vi "Lab Panel V4.86.vi"() -> ()   [LabVIEW 2013] (continued)
        }
        frame #9 {
          # "check network directory valid"
          n212 = while {
            stop <- w260 continue-if-true
            w258 = TRUE
            n213 = local read "Network Directory"() -> (w262:path)
            n214 = property on="Tab Control 2" class="TabCtl (strict)"("Value"=5) -> ()  [unwired: 2 in, 2 out]
            n215 = File/Directory Info(path=w262) -> (error out=w263:errorcluster)  [unwired: 1 in, 6 out]
            n216 = Unbundle(w263) -> ("status"=w260:bool)  [unwired: 2 out]
            n217 = case shown="True" w260 {
              frame False {
                n218 = local write "Message"("") -> ()
              }
              frame True {
                "Message" <- "NETWORK DIRECTORY NOT FOUND!!!!"
              }
            }
            n219 = property on="Message" class="Str"("Text.TextColor"=u32 16711680) -> ()  [unwired: 2 in, 2 out]
            n220 = property on="Network Directory" class="Path"("Blinking"=w258) -> ()  [unwired: 2 in, 2 out]
            n221 = property on="Message" class="Str"("Blinking"=w258) -> ()  [unwired: 2 in, 2 out]
          }
        }
        frame #10 {
          w266 = FALSE
          n222 = property on="Message" class="Str"("Blinking"=w266) -> ()  [unwired: 2 in, 2 out]
          n223 = property on="Network Directory" class="Path"("Blinking"=w266) -> ()  [unwired: 2 in, 2 out]
          n224 = property on="Tab Control 2" class="TabCtl (strict)"("Value"=0) -> ()  [unwired: 2 in, 2 out]
        }
      }
    }
    frame #2 {
      n225 = node-c288("loop  delay(mS)") -> (w270:T15)  [unwired: 3 in]
      n226 = timed-loop {
        timing: w270 -> [_]
        timing-out: [_] -> w269
        i -> [w292]
        stop <- "stop" stop-if-true
        n227 = node-c288() -> ()  [unwired: 1 in, 1 out]
        n228 = global write "Global display 1.vi" "stop disp"("stop") -> ()
        n229 = local read "SELECT LAB05-2"() -> (w272:T3)
        n230 = local read "SELECT LAB05-1"() -> (w273:T3)
        n231 = local read "SELECT LAB04-2"() -> (w274:T3)
        n232 = local read "SELECT LAB03-1"() -> (w277:T3)
        n233 = local read "SELECT LAB02-2"() -> (w278:T3)
        n234 = local read "SELECT LAB01-1"() -> (w281:T3)
        n235 = local read "SELECT LAB03-2"() -> (w276:T3)
        n236 = local read "SELECT LAB01-2"() -> (w280:T3)
        n237 = local read "SELECT LAB04-1"() -> (w275:T3)
        n238 = local read "SELECT LAB02-1"() -> (w279:T3)
        n239 = local read "run lab03-2"() -> (w286:bool)
        n240 = local read "run lab04-1"() -> (w285:bool)
        n241 = local read "run lab05-1"() -> (w283:bool)
        n242 = local read "run lab04-2"() -> (w284:bool)
        n243 = local read "run lab05-2"() -> (w282:bool)
        n244 = local read "run lab03-1"() -> (w287:bool)
        n245 = local read "run lab02-2"() -> (w288:bool)
        n246 = local read "run lab02-1"() -> (w289:bool)
        n247 = local read "run lab01-1"() -> (w291:bool)
        n248 = local read "run lab01-2"() -> (w290:bool)
        n249 = stacked-sequence {
          seq-local: [_ w354 _ _ _ _ _ _ _ _ _ _ _ _ _ _ _ _ _ _ _ _] -> [_ _ _ _ _ w2146 _ _ _ _ _ _ _ _ _ _ _ _ _ _ _ _]
          seq-local: [_ w353 _ _ _ _ _ _ _ _ _ _ _ _ _ _ _ _ _ _ _ _] -> [_ _ _ _ _ w2145 _ _ _ _ _ _ _ _ _ _ _ _ _ _ _ _]
          seq-local: [_ w340 _ _ _ _ _ _ _ _ _ _ _ _ _ _ _ _ _ _ _ _] -> [_ _ _ _ _ w2144 _ _ _ _ _ _ _ _ _ _ _ _ _ _ _ _]
          seq-local: [_ w339 _ _ _ _ _ _ _ _ _ _ _ _ _ _ _ _ _ _ _ _] -> [_ _ _ _ _ w2143 _ _ _ _ _ _ _ _ _ _ _ _ _ _ _ _]
          seq-local: [_ w338 _ _ _ _ _ _ _ _ _ _ _ _ _ _ _ _ _ _ _ _] -> [_ _ _ _ _ w2142 _ _ _ _ _ _ _ _ _ _ _ _ _ _ _ _]
          seq-local: [_ w337 _ _ _ _ _ _ _ _ _ _ _ _ _ _ _ _ _ _ _ _] -> [_ _ _ _ _ w2141 _ _ _ _ _ _ _ _ _ _ _ _ _ _ _ _]
          seq-local: [_ w336 _ _ _ _ _ _ _ _ _ _ _ _ _ _ _ _ _ _ _ _] -> [_ _ _ _ _ w2140 _ _ _ _ _ _ _ _ _ _ _ _ _ _ _ _]
          seq-local: [_ w335 _ _ _ _ _ _ _ _ _ _ _ _ _ _ _ _ _ _ _ _] -> [_ _ _ _ _ w2139 _ _ _ _ _ _ _ _ _ _ _ _ _ _ _ _]
          seq-local: [_ w334 _ _ _ _ _ _ _ _ _ _ _ _ _ _ _ _ _ _ _ _] -> [_ _ _ _ _ w2138 _ _ _ _ _ _ _ _ _ _ _ _ _ _ _ _]
          seq-local: [_ w333 _ _ _ _ _ _ _ _ _ _ _ _ _ _ _ _ _ _ _ _] -> [_ _ _ _ _ w2137 _ _ _ _ _ _ _ _ _ _ _ _ _ _ _ _]
          tunnel: w291 -> [_ _ w370 w612 w1736 w2166 w2481 w2968 _ _ _ _ w3372 _ w4306 _ _ w4591 w4894 w5075 _ _]
          tunnel: w290 -> [_ _ w369 w610 w1735 w2165 w2482 w2967 _ _ _ _ w3371 _ w4304 _ _ w4590 w4893 w5073 _ _]
          tunnel: w289 -> [_ _ w368 w608 w1734 w2164 w2480 w2966 _ _ _ _ w3370 _ w4302 _ _ w4589 w4892 w5072 _ _]
          tunnel: w288 -> [_ _ w367 w606 w1733 w2163 w2479 w2965 _ _ _ _ w3369 _ w4300 _ _ w4588 w4891 w5071 _ _]
          tunnel: w287 -> [_ _ w366 w604 w1732 w2162 w2478 w2964 _ _ _ _ w3368 _ w4298 _ _ w4587 w4890 w5070 _ _]
          tunnel: w286 -> [_ _ w365 w602 w1731 w2161 w2477 w2963 _ _ _ _ w3367 _ w4296 _ _ w4586 w4889 w5069 _ _]
          tunnel: w285 -> [_ _ w364 w600 w1730 w2160 w2476 w2962 _ _ _ _ w3366 _ w4294 _ _ w4585 w4888 w5068 _ _]
          tunnel: w284 -> [_ _ w363 w598 w1729 w2159 w2475 w2961 _ _ _ _ w3365 _ w4292 _ _ w4584 w4887 w5067 _ _]
          tunnel: w283 -> [_ _ w362 w596 w1728 w2158 w2474 w2960 _ _ _ _ w3364 _ w4290 _ _ w4583 w4886 w5066 _ _]
          tunnel: w282 -> [_ _ w361 w594 w1727 w2157 w2473 w2959 _ _ _ _ w3363 _ w4288 _ _ w4582 w4885 w5065 _ _]
          tunnel: w281 -> [_ _ _ w611 w1726 w2156 _ _ _ _ _ _ _ _ w4308 _ _ _ _ _ w5389 _]
          tunnel: w280 -> [_ _ _ w609 w1725 w2155 _ _ _ _ _ _ _ _ w4303 _ _ _ _ _ w5388 _]
          tunnel: w279 -> [_ _ _ w607 w1724 w2154 _ _ _ _ _ _ _ _ w4301 _ _ _ _ _ w5387 _]
          tunnel: w278 -> [_ _ _ w605 w1723 w2153 _ _ _ _ _ _ _ _ w4299 _ _ _ _ _ w5386 _]
          tunnel: w277 -> [_ _ _ w603 w1722 w2152 _ _ _ _ _ _ _ _ w4297 _ _ _ _ _ w5385 _]
          tunnel: w276 -> [_ _ _ w601 w1721 w2151 _ _ _ _ _ _ _ _ w4295 _ _ _ _ _ w5384 _]
          tunnel: w275 -> [_ _ _ w599 w1720 w2150 _ _ _ _ _ _ _ _ w4293 _ _ _ _ _ w5383 _]
          tunnel: w274 -> [_ _ _ w597 w1719 w2149 _ _ _ _ _ _ _ _ w4291 _ _ _ _ _ w5382 _]
          tunnel: w273 -> [_ _ _ w595 w1718 w2148 _ _ _ _ _ _ _ _ w4289 _ _ _ _ _ w5381 _]
          tunnel: w272 -> [_ _ _ w593 w1717 w2147 _ _ _ _ _ _ _ _ w4287 _ _ _ _ _ w5380 _]
          frame #0 {
            w296 = FALSE
            w301 = 0.5
            # "set up cycle control"
            n250 = local read "jig cycle"() -> (w300:dbl)
            n251 = Divide(x="JIG ON TIME (S)", y=w301) -> (x/y=→"on loops":dbl)
            n252 = Divide(x="JIG OFF TIME (S)", y=w301) -> (x/y=→"off loops":dbl)
            n253 = Increment(x=w300) -> (x+1=w299:dbl)
            n254 = local write "TEMP"(w296) -> ()
            n255 = local write "AI"(w296) -> ()
            n256 = local write "jig cycle"(w299) -> ()
            n257 = event shown="[1] \"ADMIN\": Value Change" {
              selector: _ -> [_ _]
              dyn-events: _ -> [_ _]
              timeout: 10 -> [_ _]
              event Timeout {
                n258 = event-data() -> ()  [unwired: 1 in, 3 out]
              }
              event "ADMIN": Value Change {
                n259 = event-data() -> ()  [unwired: 1 in, 6 out]
                n260 = stacked-sequence {
                  seq-local: [_ w305 _] -> [_ _ w306]
                  frame #0 {
                    n261 = global write "Global 1.vi" "password"("9999") -> ()
                  }
                  frame #1 {
                    n262 = call "sub vi - password 1.vi"() -> ("RESULT"=w305:bool)  [unwired: 11 in]
                  }
                  frame #2 {
                    w308 = FALSE
                    n263 = property on="Tab Control 2" class="TabCtl (strict)"() -> ("Pages"=w312:refnum<vi>[])  [unwired: 2 in, 2 out]
                    n264 = Select(t=TRUE, s=w306, f=w308) -> (s? t:f=w307:bool)
                    n265 = Index Array(array=w312, index=9) -> (element=w310:refnum<vi>)
                    n266 = property class="Page"(reference=w310, "PageVis"=w307) -> ()  [unwired: 1 in, 2 out]
                    n267 = local write "ADMIN"(w308) -> ()
                  }
                }
              }
            }
          }
          frame #1 {
            w350 = 60.0
            # "convert temperature rise minutes to cycles"
            n268 = local read "SET LAB05-2"() -> (w314:T5)
            n269 = local read "SET LAB05-1"() -> (w316:T5)
            n270 = local read "SET LAB04-2"() -> (w318:T5)
            n271 = local read "SET LAB01-1"() -> (w332:T5)
            n272 = local read "SET LAB01-2"() -> (w330:T5)
            n273 = local read "SET LAB02-2"() -> (w326:T5)
            n274 = local read "SET LAB04-1"() -> (w320:T5)
            n275 = local read "SET LAB03-1"() -> (w324:T5)
            n276 = local read "SET LAB03-2"() -> (w322:T5)
            n277 = local read "SET LAB02-1"() -> (w328:T5)
            n278 = local read "JIG OFF TIME (S)"() -> (w355:dbl)
            n279 = local read "JIG ON TIME (S)"() -> (w356:dbl)
            n280 = Unbundle(w314) -> ("T-RISE mins"=w313:dbl)  [unwired: 4 out]
            n281 = Unbundle(w316) -> ("T-RISE mins"=w315:dbl)  [unwired: 4 out]
            n282 = Unbundle(w332) -> ("T-RISE mins"=w331:dbl)  [unwired: 4 out]
            n283 = Unbundle(w318) -> ("T-RISE mins"=w317:dbl)  [unwired: 4 out]
            n284 = Unbundle(w330) -> ("T-RISE mins"=w329:dbl)  [unwired: 4 out]
            n285 = Unbundle(w328) -> ("T-RISE mins"=w327:dbl)  [unwired: 4 out]
            n286 = Unbundle(w320) -> ("T-RISE mins"=w319:dbl)  [unwired: 4 out]
            n287 = Unbundle(w326) -> ("T-RISE mins"=w325:dbl)  [unwired: 4 out]
            n288 = Unbundle(w322) -> ("T-RISE mins"=w321:dbl)  [unwired: 4 out]
            n289 = Unbundle(w324) -> ("T-RISE mins"=w323:dbl)  [unwired: 4 out]
            n290 = Add(x=w356, y=w355) -> (x+y=w349:dbl)
            n291 = Multiply(x=w350, y=w321) -> (x*y=w345:dbl)
            n292 = Multiply(x=w350, y=w319) -> (x*y=w344:dbl)
            n293 = Multiply(x=w350, y=w317) -> (x*y=w343:dbl)
            n294 = Multiply(x=w350, y=w315) -> (x*y=w342:dbl)
            n295 = Multiply(x=w350, y=w313) -> (x*y=w341:dbl)
            n296 = Multiply(x=w350, y=w329) -> (x*y=w351:dbl)
            n297 = Multiply(x=w350, y=w323) -> (x*y=w346:dbl)
            n298 = Multiply(x=w350, y=w331) -> (x*y=w352:dbl)
            n299 = Multiply(x=w350, y=w327) -> (x*y=w348:dbl)
            n300 = Multiply(x=w350, y=w325) -> (x*y=w347:dbl)
            n301 = Divide(x=w342, y=w349) -> (x/y=w334:dbl)
            n302 = Divide(x=w343, y=w349) -> (x/y=w335:dbl)
            n303 = Divide(x=w344, y=w349) -> (x/y=w336:dbl)
            n304 = Divide(x=w341, y=w349) -> (x/y=w333:dbl)
            n305 = Divide(x=w346, y=w349) -> (x/y=w338:dbl)
            n306 = Divide(x=w352, y=w349) -> (x/y=w354:dbl)
            n307 = Divide(x=w351, y=w349) -> (x/y=w353:dbl)
            n308 = Divide(x=w348, y=w349) -> (x/y=w340:dbl)
            n309 = Divide(x=w347, y=w349) -> (x/y=w339:dbl)
            n310 = Divide(x=w345, y=w349) -> (x/y=w337:dbl)
          }
          frame #2 {
            # "control cycle loops"
            n311 = local read "JIG OFF TIME (S)"() -> (w359:dbl)
            n312 = local read "JIG ON TIME (S)"() -> (w358:dbl)
            n313 = local read "jig cycle"() -> (w372:dbl)
            n314 = local read "on loops"() -> (w374:dbl)
            n315 = local read "off loops"() -> (w373:dbl)
            n316 = Add(x=w359, y=w358) -> (x+y=w357:dbl)
            n317 = Add(x=w374, y=w373) -> (x+y=w360:dbl)
            n318 = Greater Or Equal?(x=w372, y=w360) -> (x >= y?=w371:bool)
            n319 = case shown="True" w371 {
              tunnel: w370 -> [_ w409]
              tunnel: w369 -> [_ w408]
              tunnel: w368 -> [_ w407]
              tunnel: w367 -> [_ w406]
              tunnel: w366 -> [_ w405]
              tunnel: w365 -> [_ w404]
              tunnel: w364 -> [_ w403]
              tunnel: w363 -> [_ w402]
              tunnel: w362 -> [_ w401]
              tunnel: w361 -> [_ w400]
              tunnel: w357 -> [_ w399]
              frame False {
              }
              frame True {
                # "increment cycle value and convert cycles to minutes for temp rise"
                n320 = local read "Temp Loops"() -> (w376:dbl)
                n321 = local read "JIG RELAY CYCLES"() -> (w398:T7)
                n322 = Increment(x=w376) -> (x+1=w375:dbl)
                n323 = local write "Temp Loops"(w375) -> ()
                n324 = Unbundle By Name(w398) -> ("LAB01-1"=w396:dbl, "LAB01-2"=w394:dbl, "LAB02-1"=w392:dbl, "LAB02-2"=w390:dbl, "LAB03-1"=w388:dbl, "LAB03-2"=w386:dbl, "LAB04-1"=w384:dbl, "LAB04-2"=w382:dbl, "LAB05-1"=w380:dbl, "LAB05-2"=w378:dbl)
                n325 = stacked-sequence {
                  tunnel: w409 -> [w421 _ _ _ _ _ _ _ _ _]
                  tunnel: w408 -> [_ w438 _ _ _ _ _ _ _ _]
                  tunnel: w407 -> [_ _ w455 _ _ _ _ _ _ _]
                  tunnel: w406 -> [_ _ _ w472 _ _ _ _ _ _]
                  tunnel: w405 -> [_ _ _ _ w489 _ _ _ _ _]
                  tunnel: w404 -> [_ _ _ _ _ w506 _ _ _ _]
                  tunnel: w403 -> [_ _ _ _ _ _ w523 _ _ _]
                  tunnel: w402 -> [_ _ _ _ _ _ _ w540 _ _]
                  tunnel: w401 -> [_ _ _ _ _ _ _ _ w557 _]
                  tunnel: w400 -> [_ _ _ _ _ _ _ _ _ w574]
                  tunnel: w399 -> [w418 w435 w452 w469 w486 w503 w520 w537 w554 w571]
                  tunnel: w396 -> [w412 _ _ _ _ _ _ _ _ _]
                  tunnel: [w411 _ _ _ _ _ _ _ _ _] -> w395
                  tunnel: w394 -> [_ w429 _ _ _ _ _ _ _ _]
                  tunnel: [_ w428 _ _ _ _ _ _ _ _] -> w393
                  tunnel: w392 -> [_ _ w446 _ _ _ _ _ _ _]
                  tunnel: [_ _ w445 _ _ _ _ _ _ _] -> w391
                  tunnel: w390 -> [_ _ _ w463 _ _ _ _ _ _]
                  tunnel: [_ _ _ w462 _ _ _ _ _ _] -> w389
                  tunnel: w388 -> [_ _ _ _ w480 _ _ _ _ _]
                  tunnel: [_ _ _ _ w479 _ _ _ _ _] -> w387
                  tunnel: w386 -> [_ _ _ _ _ w497 _ _ _ _]
                  tunnel: [_ _ _ _ _ w496 _ _ _ _] -> w385
                  tunnel: w384 -> [_ _ _ _ _ _ w514 _ _ _]
                  tunnel: [_ _ _ _ _ _ w513 _ _ _] -> w383
                  tunnel: w382 -> [_ _ _ _ _ _ _ w531 _ _]
                  tunnel: [_ _ _ _ _ _ _ w530 _ _] -> w381
                  tunnel: w380 -> [_ _ _ _ _ _ _ _ w548 _]
                  tunnel: [_ _ _ _ _ _ _ _ w547 _] -> w379
                  tunnel: w378 -> [_ _ _ _ _ _ _ _ _ w565]
                  tunnel: [_ _ _ _ _ _ _ _ _ w564] -> w377
                  frame #0 {
                    n326 = local read "DISP LAB01-1"() -> (w416:T4)
                    n327 = Unbundle(w416) -> ("CYCLE"=w417:dbl)  [unwired: 2 out]
                    n328 = case shown="True" w421 {
                      tunnel: w417 -> [w423 w427]
                      tunnel: [w423 w426] -> w415
                      tunnel: w412 -> [w422 w425]
                      tunnel: [w422 w424] -> w411
                      frame False {
                      }
                      frame True {
                        n329 = Increment(x=w425) -> (x+1=w424:dbl)
                        n330 = Increment(x=w427) -> (x+1=w426:dbl)
                      }
                    }
                    n331 = Multiply(x=w415, y=w418) -> (x*y=w419:dbl)
                    n332 = Divide(x=w419, y=60.0) -> (x/y=w414:dbl)
                    n333 = Bundle(cluster=w416, "CYCLE"=w415, "MINS"=w414) -> (w413:T4)  [unwired: 1 in]
                    n334 = local write "DISP LAB01-1"(w413) -> ()
                  }
                  frame #1 {
                    n335 = local read "DISP LAB01-2"() -> (w433:T4)
                    n336 = Unbundle(w433) -> ("CYCLE"=w434:dbl)  [unwired: 2 out]
                    n337 = case shown="True" w438 {
                      tunnel: w434 -> [w440 w444]
                      tunnel: [w440 w443] -> w431
                      tunnel: w429 -> [w439 w442]
                      tunnel: [w439 w441] -> w428
                      frame False {
                      }
                      frame True {
                        n338 = Increment(x=w442) -> (x+1=w441:dbl)
                        n339 = Increment(x=w444) -> (x+1=w443:dbl)
                      }
                    }
                    n340 = Multiply(x=w431, y=w435) -> (x*y=w436:dbl)
                    n341 = Divide(x=w436, y=60.0) -> (x/y=w430:dbl)
                    n342 = Bundle(cluster=w433, "CYCLE"=w431, "MINS"=w430) -> (w432:T4)  [unwired: 1 in]
                    n343 = local write "DISP LAB01-2"(w432) -> ()
                  }
                  frame #2 {
                    n344 = local read "DISP LAB02-1"() -> (w450:T4)
                    n345 = Unbundle(w450) -> ("CYCLE"=w451:dbl)  [unwired: 2 out]
                    n346 = case shown="True" w455 {
                      tunnel: [w457 w461] -> w448
                      tunnel: w451 -> [w457 w460]
                      tunnel: w446 -> [w456 w459]
                      tunnel: [w456 w458] -> w445
                      frame False {
                      }
                      frame True {
                        n347 = Increment(x=w459) -> (x+1=w458:dbl)
                        n348 = Increment(x=w460) -> (x+1=w461:dbl)
                      }
                    }
                    n349 = Multiply(x=w448, y=w452) -> (x*y=w453:dbl)
                    n350 = Divide(x=w453, y=60.0) -> (x/y=w447:dbl)
                    n351 = Bundle(cluster=w450, "CYCLE"=w448, "MINS"=w447) -> (w449:T4)  [unwired: 1 in]
                    n352 = local write "DISP LAB02-1"(w449) -> ()
                  }
                  frame #3 {
                    n353 = local read "DISP LAB02-2"() -> (w467:T4)
                    n354 = Unbundle(w467) -> ("CYCLE"=w468:dbl)  [unwired: 2 out]
                    n355 = case shown="True" w472 {
                      tunnel: [w474 w478] -> w466
                      tunnel: w468 -> [w474 w477]
                      tunnel: w463 -> [w473 w476]
                      tunnel: [w473 w475] -> w462
                      frame False {
                      }
                      frame True {
                        n356 = Increment(x=w476) -> (x+1=w475:dbl)
                        n357 = Increment(x=w477) -> (x+1=w478:dbl)
                      }
                    }
                    n358 = Multiply(x=w466, y=w469) -> (x*y=w470:dbl)
                    n359 = Divide(x=w470, y=60.0) -> (x/y=w465:dbl)
                    n360 = Bundle(cluster=w467, "CYCLE"=w466, "MINS"=w465) -> (w464:T4)  [unwired: 1 in]
                    n361 = local write "DISP LAB02-2"(w464) -> ()
                  }
                  frame #4 {
                    n362 = local read "DISP LAB03-1"() -> (w484:T4)
                    n363 = Unbundle(w484) -> ("CYCLE"=w485:dbl)  [unwired: 2 out]
                    n364 = case shown="True" w489 {
                      tunnel: [w491 w495] -> w481
                      tunnel: w485 -> [w491 w494]
                      tunnel: w480 -> [w490 w493]
                      tunnel: [w490 w492] -> w479
                      frame False {
                      }
                      frame True {
                        n365 = Increment(x=w493) -> (x+1=w492:dbl)
                        n366 = Increment(x=w494) -> (x+1=w495:dbl)
                      }
                    }
                    n367 = Multiply(x=w481, y=w486) -> (x*y=w487:dbl)
                    n368 = Divide(x=w487, y=60.0) -> (x/y=w482:dbl)
                    n369 = Bundle(cluster=w484, "CYCLE"=w481, "MINS"=w482) -> (w483:T4)  [unwired: 1 in]
                    n370 = local write "DISP LAB03-1"(w483) -> ()
                  }
                  frame #5 {
                    n371 = local read "DISP LAB03-2"() -> (w501:T4)
                    n372 = Unbundle(w501) -> ("CYCLE"=w502:dbl)  [unwired: 2 out]
                    n373 = case shown="True" w506 {
                      tunnel: [w508 w512] -> w500
                      tunnel: w502 -> [w508 w511]
                      tunnel: w497 -> [w507 w510]
                      tunnel: [w507 w509] -> w496
                      frame False {
                      }
                      frame True {
                        n374 = Increment(x=w510) -> (x+1=w509:dbl)
                        n375 = Increment(x=w511) -> (x+1=w512:dbl)
                      }
                    }
                    n376 = Multiply(x=w500, y=w503) -> (x*y=w504:dbl)
                    n377 = Divide(x=w504, y=60.0) -> (x/y=w499:dbl)
                    n378 = Bundle(cluster=w501, "CYCLE"=w500, "MINS"=w499) -> (w498:T4)  [unwired: 1 in]
                    n379 = local write "DISP LAB03-2"(w498) -> ()
                  }
                  frame #6 {
                    n380 = local read "DISP LAB04-1"() -> (w518:T4)
                    n381 = Unbundle(w518) -> ("CYCLE"=w519:dbl)  [unwired: 2 out]
                    n382 = case shown="True" w523 {
                      tunnel: [w525 w529] -> w516
                      tunnel: w519 -> [w525 w528]
                      tunnel: w514 -> [w524 w527]
                      tunnel: [w524 w526] -> w513
                      frame False {
                      }
                      frame True {
                        n383 = Increment(x=w527) -> (x+1=w526:dbl)
                        n384 = Increment(x=w528) -> (x+1=w529:dbl)
                      }
                    }
                    n385 = Multiply(x=w516, y=w520) -> (x*y=w521:dbl)
                    n386 = Divide(x=w521, y=60.0) -> (x/y=w515:dbl)
                    n387 = Bundle(cluster=w518, "CYCLE"=w516, "MINS"=w515) -> (w517:T4)  [unwired: 1 in]
                    n388 = local write "DISP LAB04-1"(w517) -> ()
                  }
                  frame #7 {
                    n389 = local read "DISP LAB04-2"() -> (w535:T4)
                    n390 = Unbundle(w535) -> ("CYCLE"=w536:dbl)  [unwired: 2 out]
                    n391 = case shown="True" w540 {
                      tunnel: [w542 w546] -> w533
                      tunnel: w536 -> [w542 w545]
                      tunnel: w531 -> [w541 w544]
                      tunnel: [w541 w543] -> w530
                      frame False {
                      }
                      frame True {
                        n392 = Increment(x=w544) -> (x+1=w543:dbl)
                        n393 = Increment(x=w545) -> (x+1=w546:dbl)
                      }
                    }
                    n394 = Multiply(x=w533, y=w537) -> (x*y=w539:dbl)
                    n395 = Divide(x=w539, y=60.0) -> (x/y=w532:dbl)
                    n396 = Bundle(cluster=w535, "CYCLE"=w533, "MINS"=w532) -> (w534:T4)  [unwired: 1 in]
                    n397 = local write "DISP LAB04-2"(w534) -> ()
                  }
                  frame #8 {
                    n398 = local read "DISP LAB05-1"() -> (w552:T4)
                    n399 = Unbundle(w552) -> ("CYCLE"=w553:dbl)  [unwired: 2 out]
                    n400 = case shown="True" w557 {
                      tunnel: [w559 w563] -> w550
                      tunnel: w553 -> [w559 w562]
                      tunnel: w548 -> [w558 w561]
                      tunnel: [w558 w560] -> w547
                      frame False {
                      }
                      frame True {
                        n401 = Increment(x=w561) -> (x+1=w560:dbl)
                        n402 = Increment(x=w562) -> (x+1=w563:dbl)
                      }
                    }
                    n403 = Multiply(x=w550, y=w554) -> (x*y=w555:dbl)
                    n404 = Divide(x=w555, y=60.0) -> (x/y=w549:dbl)
                    n405 = Bundle(cluster=w552, "CYCLE"=w550, "MINS"=w549) -> (w551:T4)  [unwired: 1 in]
                    n406 = local write "DISP LAB05-1"(w551) -> ()
                  }
                  frame #9 {
                    n407 = local read "DISP LAB05-2"() -> (w570:T4)
                    n408 = Unbundle(w570) -> ("CYCLE"=w569:dbl)  [unwired: 2 out]
                    n409 = case shown="True" w574 {
                      tunnel: [w576 w580] -> w568
                      tunnel: w569 -> [w576 w579]
                      tunnel: w565 -> [w575 w578]
                      tunnel: [w575 w577] -> w564
                      frame False {
                      }
                      frame True {
                        n410 = Increment(x=w578) -> (x+1=w577:dbl)
                        n411 = Increment(x=w579) -> (x+1=w580:dbl)
                      }
                    }
                    n412 = Multiply(x=w568, y=w571) -> (x*y=w572:dbl)
                    n413 = Divide(x=w572, y=60.0) -> (x/y=w567:dbl)
                    n414 = Bundle(cluster=w570, "CYCLE"=w568, "MINS"=w567) -> (w566:T4)  [unwired: 1 in]
                    n415 = local write "DISP LAB05-2"(w566) -> ()
                  }
                }
                n416 = local write "jig cycle"(0) -> ()
                n417 = Bundle By Name(cluster=w398, "LAB01-1"=w395, "LAB01-2"=w393, "LAB02-1"=w391, "LAB02-2"=w389, "LAB03-1"=w387, "LAB03-2"=w385, "LAB04-1"=w383, "LAB04-2"=w381, "LAB05-1"=w379, "LAB05-2"=w377) -> (w397:T7)
                n418 = local write "JIG RELAY CYCLES"(w397) -> ()
              }
            }
          }
          frame #3 {
            # "START & STOP test RUN switch change, start test if true and stop test if false"
            n419 = Get Date/Time In Seconds() -> (seconds since 1Jan1904=w591:timestamp)
            n420 = local read "C drive data root dir"() -> (w584:path)
            n421 = Format Date/Time String(time format string (%c)="%b\\%a%d", seconds (now)=w591) -> (date/time string=w615:string)  [unwired: 1 in]
            n422 = Format Date/Time String(time format string (%c)="%H%M", seconds (now)=w591) -> (date/time string=w613:string)  [unwired: 1 in]
            n423 = Format Date/Time String(time format string (%c)="LabPanel%Y", seconds (now)=w591) -> (date/time string=w590:string)  [unwired: 1 in]
            n424 = Path To String(path=w584) -> (string=w587:string)
            n425 = global write "Global 1.vi" "C drive root path"(w584) -> ()
            n426 = Concatenate Strings(w587, "\\") -> (w585:string)
            n427 = event shown="[1] \"RUN LAB01-1\": Value Change" {
              selector: _ -> [_ _ _ _ _ _ _ _ _ _ _]
              dyn-events: _ -> [_ _ _ _ _ _ _ _ _ _ _]
              timeout: 10 -> [_ _ _ _ _ _ _ _ _ _ _]
              tunnel: w585 -> [_ w626 w736 w846 w956 w1066 w1176 w1286 w1396 w1506 w1616]
              tunnel: w615 -> [_ w625 w735 w845 w955 w1065 w1175 w1285 w1395 w1505 w1615]
              tunnel: w613 -> [_ w623 w734 w844 w954 w1064 w1174 w1284 w1394 w1504 w1614]
              tunnel: w611 -> [_ w624 _ _ _ _ _ _ _ _ _]
              tunnel: w612 -> [_ _ _ _ _ _ _ _ _ _ _]
              tunnel: w610 -> [_ _ _ _ _ _ _ _ _ _ _]
              tunnel: w609 -> [_ _ w733 _ _ _ _ _ _ _ _]
              tunnel: w608 -> [_ _ _ _ _ _ _ _ _ _ _]
              tunnel: w607 -> [_ _ _ w843 _ _ _ _ _ _ _]
              tunnel: w606 -> [_ _ _ _ _ _ _ _ _ _ _]
              tunnel: w605 -> [_ _ _ _ w953 _ _ _ _ _ _]
              tunnel: w604 -> [_ _ _ _ _ _ _ _ _ _ _]
              tunnel: w603 -> [_ _ _ _ _ w1063 _ _ _ _ _]
              tunnel: w602 -> [_ _ _ _ _ _ _ _ _ _ _]
              tunnel: w601 -> [_ _ _ _ _ _ w1173 _ _ _ _]
              tunnel: w600 -> [_ _ _ _ _ _ _ _ _ _ _]
              tunnel: w599 -> [_ _ _ _ _ _ _ w1283 _ _ _]
              tunnel: w598 -> [_ _ _ _ _ _ _ _ _ _ _]
              tunnel: w597 -> [_ _ _ _ _ _ _ _ w1393 _ _]
              tunnel: w596 -> [_ _ _ _ _ _ _ _ _ _ _]
              tunnel: w595 -> [_ _ _ _ _ _ _ _ _ w1503 _]
              tunnel: w594 -> [_ _ _ _ _ _ _ _ _ _ _]
              tunnel: w593 -> [_ _ _ _ _ _ _ _ _ _ w1613]
              tunnel: w590 -> [_ w622 w732 w842 w952 w1062 w1172 w1282 w1392 w1502 w1612]
              tunnel: [_ w621 w731 w841 w951 w1061 w1171 w1281 w1391 w1501 w1611] -> w588
              tunnel: "RESET CYCLES TO ZERO?" -> [_ w619 w729 w839 w949 w1059 w1169 w1279 w1389 w1499 w1609]
              tunnel: "YES" -> [_ w618 w728 w838 w948 w1058 w1168 w1278 w1388 w1498 w1608]
              tunnel: "NO" -> [_ w617 w727 w837 w947 w1057 w1167 w1277 w1387 w1497 w1607]
              event Timeout {
                n428 = event-data() -> ()  [unwired: 1 in, 3 out]
              }
              event "RUN LAB01-1": Value Change {
                n429 = event-data() -> ("NewVal"=w620:bool)  [unwired: 1 in, 5 out]
                n430 = local write "run lab01-1"(w620) -> ()
                n431 = case shown="True" w620 {
                  tunnel: w626 -> [_ w662]
                  tunnel: w625 -> [_ w661]
                  tunnel: w624 -> [w628 w660]
                  tunnel: w623 -> [_ w659]
                  tunnel: w622 -> [_ w658]
                  tunnel: [w627 w657] -> w621
                  tunnel: w619 -> [_ w656]
                  tunnel: w618 -> [_ w655]
                  tunnel: w617 -> [_ w654]
                  frame False {
                    # "stop test"
                    n432 = stacked-sequence {
                      tunnel: w628 -> [_ w640 _]
                      tunnel: [_ w632 _] -> w627
                      frame #0 {
                        n433 = local read "DISP LAB01-1"() -> (w631:T4)
                        n434 = Bundle(cluster=w631, "STATUS"="STOP") -> (w629:T4)  [unwired: 2 in]
                        n435 = local write "DISP LAB01-1"(w629) -> ()
                      }
                      frame #1 {
                        n436 = local read "DISP LAB01-1"() -> (w639:T4)
                        n437 = Unbundle(w639) -> ("CYCLE"=w637:dbl, "MINS"=w638:dbl)  [unwired: 1 out]
                        n438 = case shown="\"CYCLE TEST\"" w640 {
                          tunnel: w638 -> [_ _ w647]
                          tunnel: w637 -> [w645 w646 _]
                          tunnel: [w645 w646 w647] -> w636
                          frame "CHART TEST", Default {
                          }
                          frame "CYCLE TEST" {
                          }
                          frame "T-RISE TEST" {
                          }
                        }
                        n439 = local read "TDMS LAB01-1"() -> (w644:refnum<k34>)
                        n440 = Build Array("STOPPED") -> (w641:string[])
                        n441 = Build Array(w636) -> (w635:dbl[])
                        n442 = TDMS Write(0:w644, 5:"TEST RESULT", 7:w641, 9:w635) -> (4:w633:refnum<k34>, 15:w634:errorcluster)  [unwired: 2 in, 2 out]
                        n443 = TDMS Close(8:w634, 11:w633) -> (0:w632:errorcluster)  [unwired: 1 out]
                      }
                      frame #2 {
                        n444 = stacked-sequence {
                          tunnel: "LAB01-1" -> [w650 w652]
                          frame #0 {
                            n445 = call "sub vi - defrag tdms v1.vi"("panel id"=w650) -> ("error out"=w649:errorcluster)  [unwired: 10 in]
                            n446 = local write "data file error"(w649) -> ()
                          }
                          frame #1 {
                            n447 = call "Save data file to network drive v2.vi"("panel id"=w652) -> ("network file save error"=w651:errorcluster)  [unwired: 9 in, 1 out]
                            n448 = local write "RESULT LAB01-1"(FALSE) -> ()
                            n449 = local write "data file error"(w651) -> ()
                          }
                        }
                      }
                    }
                  }
                  frame True {
                    # "start new test and create test file"
                    n450 = stacked-sequence {
                      seq-local: [w663 _ _ _ _] -> [_ w684 _ _ _]
                      tunnel: w662 -> [w668 _ _ _ _]
                      tunnel: w661 -> [w664 _ _ _ _]
                      tunnel: w660 -> [w678 _ _ _ _]
                      tunnel: w659 -> [w671 _ _ _ _]
                      tunnel: w658 -> [w666 _ _ _ _]
                      tunnel: [_ w685 _ _ _] -> w657
                      tunnel: w656 -> [_ _ _ w706 _]
                      tunnel: w655 -> [_ _ _ w716 _]
                      tunnel: w654 -> [_ _ _ w715 _]
                      frame #0 {
                        w665 = "\\"
                        n451 = case shown="\"CHART TEST\", Default" w678 {
                          tunnel: ["L01-1-CHART TEST-" "L01-1-CYCLE TEST-" "L01-1-T-RISE TEST-"] -> w674
                          frame "CHART TEST", Default {
                          }
                          frame "CYCLE TEST" {
                          }
                          frame "T-RISE TEST" {
                          }
                        }
                        n452 = local read "SET LAB01-1"() -> (w673:T5)
                        n453 = Unbundle(w673) -> ("DESCRIPTION"=w672:string)  [unwired: 4 out]
                        n454 = Concatenate Strings(w668, "\\", w666, w665, w664, w665) -> (w675:string)
                        n455 = String To Path(string=w675) -> (path=w677:path)
                        n456 = Concatenate Strings(w675, w674, w672, "-", w671, ".tdms") -> (w663:string)
                        n457 = Create Folder(path (use dialog)=w677) -> (error out=w676:errorcluster)  [unwired: 2 in, 2 out]
                        n458 = call <vilib>:"Clear Errors.vi"("error in (no error)"=w676) -> ()  [unwired: 6 in, 1 out]
                        n459 = global write "Global 1.vi" "LAB01-1 FILE"(w663) -> ()
                      }
                      frame #1 {
                        (unwired) FALSE
                        n460 = String To Path(string=w684) -> (path=w682:path)
                        n461 = TDMS Open(6:FALSE, 10:T18."create or replace" ("operation (0:open)"), 11:w682) -> (0:w685:errorcluster, 3:→"TDMS LAB01-1":refnum<k34>)  [unwired: 4 in]
                      }
                      frame #2 {
                        n462 = local read "TDMS LAB01-1"() -> (w704:refnum<k34>)
                        n463 = local read "SET LAB01-1"() -> (w693:T5)
                        n464 = Build Array("Testers Name", "Description", "Set Test Cycles", "T-Rise minutes", "T-Rise Deg C") -> (w694:string[])
                        n465 = Unbundle(w693) -> ("NAME"=w692:string, "DESCRIPTION"=w691:string, "CYCLES"=w690:dbl, "T-RISE mins"=w689:dbl, "T-RISE deg C"=w688:dbl)
                        n466 = Number To Decimal String(number=w690) -> (decimal integer string=w703:string)  [unwired: 1 in]
                        n467 = Number To Decimal String(number=w689) -> (decimal integer string=w702:string)  [unwired: 1 in]
                        n468 = Number To Decimal String(number=w688) -> (decimal integer string=w701:string)  [unwired: 1 in]
                        n469 = Build Array(w692, w691, w703, w702, w701) -> (w700:string[])
                        n470 = TDMS Set Properties(5:w700, 7:w694, 11:w704) -> ()  [unwired: 3 in, 4 out]
                      }
                      frame #3 {
                        n471 = local read "DISP LAB01-1"() -> (w714:T4)
                        n472 = Concatenate Strings("LAB01-1  ", w706) -> (w705:string)
                        n473 = Two Button Dialog(message=w705, 1:w715, 2:w716) -> (T button?=w708:bool)
                        n474 = case shown="True" w708 {
                          tunnel: w714 -> [w719 w720]
                          tunnel: [w719 w720] -> w713
                          tunnel: [w718 w721] -> w712
                          tunnel: [w717 w721] -> w711
                          frame False {
                            n475 = Unbundle(w719) -> ("CYCLE"=w718:dbl, "MINS"=w717:dbl)  [unwired: 1 out]
                          }
                          frame True {
                            w721 = 0.0
                          }
                        }
                        n476 = Bundle(cluster=w713, "CYCLE"=w712, "MINS"=w711, "STATUS"="RUN") -> (w710:T4)
                        n477 = local write "DISP LAB01-1"(w710) -> ()
                      }
                      frame #4 {
                        n478 = local read "SIG LAB01-1"() -> (w724:T2)
                        n479 = local read "TEMP START LAB01-1"() -> (w726:cluster{"TL":dbl, "TN":dbl})
                        n480 = Unbundle(w724) -> ("Tmp Live"=w723:dbl, "Tmp Neut"=w722:dbl)  [unwired: 3 out]
                        n481 = Bundle(cluster=w726, "TL"=w723, "TN"=w722) -> (w725:cluster{"TL":dbl, "TN":dbl})
                        n482 = local write "TEMP START LAB01-1"(w725) -> ()
                      }
                    }
                  }
                }
              }
              event "RUN LAB01-2": Value Change {
                n483 = event-data() -> ("NewVal"=w730:bool)  [unwired: 1 in, 5 out]
                n484 = local write "run lab01-2"(w730) -> ()
                n485 = case shown="True" w730 {
                  tunnel: w736 -> [_ w772]
                  tunnel: w735 -> [_ w771]
                  tunnel: w733 -> [w738 w770]
                  tunnel: w734 -> [_ w769]
                  tunnel: w732 -> [_ w768]
                  tunnel: [w737 w767] -> w731
                  tunnel: w729 -> [_ w766]
                  tunnel: w728 -> [_ w765]
                  tunnel: w727 -> [_ w764]
                  frame False {
                    # "stop test"
                    n486 = stacked-sequence {
                      tunnel: w738 -> [w747 _]
                      tunnel: [w739 _] -> w737
                      frame #0 {
                        n487 = local read "DISP LAB01-2"() -> (w746:T4)
                        n488 = Unbundle(w746) -> ("CYCLE"=w744:dbl, "MINS"=w745:dbl)  [unwired: 1 out]
                        n489 = case shown="\"CHART TEST\", Default" w747 {
                          tunnel: w745 -> [_ _ w754]
                          tunnel: w744 -> [w752 w753 _]
                          tunnel: [w752 w753 w754] -> w743
                          frame "CHART TEST", Default {
                          }
                          frame "CYCLE TEST" {
                          }
                          frame "T-RISE TEST" {
                          }
                        }
                        n490 = local read "TDMS LAB01-2"() -> (w751:refnum<k34>)
                        n491 = Build Array("STOPPED") -> (w748:string[])
                        n492 = Build Array(w743) -> (w742:dbl[])
                        n493 = TDMS Write(0:w751, 5:"TEST RESULT", 7:w748, 9:w742) -> (4:w740:refnum<k34>, 15:w741:errorcluster)  [unwired: 2 in, 2 out]
                        n494 = TDMS Close(8:w741, 11:w740) -> (0:w739:errorcluster)  [unwired: 1 out]
                      }
                      frame #1 {
                        n495 = local read "DISP LAB01-2"() -> (w758:T4)
                        n496 = stacked-sequence {
                          tunnel: "LAB01-2" -> [w760 w762]
                          frame #0 {
                            n497 = call "sub vi - defrag tdms v1.vi"("panel id"=w760) -> ("error out"=w759:errorcluster)  [unwired: 10 in]
                            n498 = local write "data file error"(w759) -> ()
                          }
                          frame #1 {
                            n499 = call "Save data file to network drive v2.vi"("panel id"=w762) -> ("network file save error"=w761:errorcluster)  [unwired: 9 in, 1 out]
                            n500 = local write "RESULT LAB01-2"(FALSE) -> ()
                            n501 = local write "data file error"(w761) -> ()
                          }
                        }
                        n502 = Bundle(cluster=w758, "STATUS"="STOP") -> (w756:T4)  [unwired: 2 in]
                        n503 = local write "DISP LAB01-2"(w756) -> ()
                      }
                    }
                  }
                  frame True {
                    # "start new test and create test file"
                    n504 = stacked-sequence {
                      seq-local: [w773 _ _ _ _] -> [_ w797 _ _ _]
                      tunnel: w772 -> [w778 _ _ _ _]
                      tunnel: w771 -> [w775 _ _ _ _]
                      tunnel: w770 -> [w788 _ _ _ _]
                      tunnel: w769 -> [w781 _ _ _ _]
                      tunnel: w768 -> [w776 _ _ _ _]
                      tunnel: [_ w792 _ _ _] -> w767
                      tunnel: w766 -> [_ _ _ w819 _]
                      tunnel: w765 -> [_ _ _ w818 _]
                      tunnel: w764 -> [_ _ _ w817 _]
                      frame #0 {
                        w774 = "\\"
                        n505 = local read "SET LAB01-2"() -> (w783:T5)
                        n506 = case shown="\"CYCLE TEST\"" w788 {
                          tunnel: ["L01-2-CHART TEST-" "L01-2-CYCLE TEST-" "L01-2-T-RISE TEST-"] -> w784
                          frame "CHART TEST", Default {
                          }
                          frame "CYCLE TEST" {
                          }
                          frame "T-RISE TEST" {
                          }
                        }
                        n507 = Unbundle(w783) -> ("DESCRIPTION"=w782:string)  [unwired: 4 out]
                        n508 = Concatenate Strings(w778, "\\", w776, w774, w775, w774) -> (w785:string)
                        n509 = String To Path(string=w785) -> (path=w787:path)
                        n510 = Concatenate Strings(w785, w784, w782, "-", w781, ".tdms") -> (w773:string)
                        n511 = Create Folder(path (use dialog)=w787) -> (error out=w786:errorcluster)  [unwired: 2 in, 2 out]
                        n512 = global write "Global 1.vi" "LAB01-2 FILE"(w773) -> ()
                        n513 = call <vilib>:"Clear Errors.vi"("error in (no error)"=w786) -> ()  [unwired: 6 in, 1 out]
                      }
                      frame #1 {
                        (unwired) FALSE
                        n514 = String To Path(string=w797) -> (path=w793:path)
                        n515 = TDMS Open(6:FALSE, 10:T18."create or replace" ("operation (0:open)"), 11:w793) -> (0:w792:errorcluster, 3:→"TDMS LAB01-2":refnum<k34>)  [unwired: 4 in]
                      }
                      frame #2 {
                        n516 = local read "SET LAB01-2"() -> (w803:T5)
                        n517 = local read "TDMS LAB01-2"() -> (w814:refnum<k34>)
                        n518 = Build Array("Testers Name", "Description", "Set Test Cycles", "T-Rise minutes", "T-Rise Deg C") -> (w804:string[])
                        n519 = Unbundle(w803) -> ("NAME"=w802:string, "DESCRIPTION"=w801:string, "CYCLES"=w800:dbl, "T-RISE mins"=w799:dbl, "T-RISE deg C"=w798:dbl)
                        n520 = Number To Decimal String(number=w800) -> (decimal integer string=w813:string)  [unwired: 1 in]
                        n521 = Number To Decimal String(number=w799) -> (decimal integer string=w812:string)  [unwired: 1 in]
                        n522 = Number To Decimal String(number=w798) -> (decimal integer string=w811:string)  [unwired: 1 in]
                        n523 = Build Array(w802, w801, w813, w812, w811) -> (w810:string[])
                        n524 = TDMS Set Properties(5:w810, 7:w804, 11:w814) -> ()  [unwired: 3 in, 4 out]
                      }
                      frame #3 {
                        n525 = local read "DISP LAB01-2"() -> (w816:T4)
                        n526 = Concatenate Strings("LAB01-2  ", w819) -> (w820:string)
                        n527 = Two Button Dialog(message=w820, 1:w817, 2:w818) -> (T button?=w822:bool)
                        n528 = case shown="True" w822 {
                          tunnel: w816 -> [w829 w830]
                          tunnel: [w829 w830] -> w826
                          tunnel: [w828 w831] -> w825
                          tunnel: [w827 w831] -> w824
                          frame False {
                            n529 = Unbundle(w829) -> ("CYCLE"=w828:dbl, "MINS"=w827:dbl)  [unwired: 1 out]
                          }
                          frame True {
                            w831 = 0.0
                          }
                        }
                        n530 = Bundle(cluster=w826, "CYCLE"=w825, "MINS"=w824, "STATUS"="RUN") -> (w815:T4)
                        n531 = local write "DISP LAB01-2"(w815) -> ()
                      }
                      frame #4 {
                        n532 = local read "SIG LAB01-2"() -> (w834:T2)
                        n533 = local read "TEMP START LAB01-2"() -> (w836:cluster{"TL":dbl, "TN":dbl})
                        n534 = Unbundle(w834) -> ("Tmp Live"=w833:dbl, "Tmp Neut"=w832:dbl)  [unwired: 3 out]
                        n535 = Bundle(cluster=w836, "TL"=w833, "TN"=w832) -> (w835:cluster{"TL":dbl, "TN":dbl})
                        n536 = local write "TEMP START LAB01-2"(w835) -> ()
                      }
                    }
                  }
                }
              }
              event "RUN LAB02-1": Value Change {
                n537 = event-data() -> ("NewVal"=w840:bool)  [unwired: 1 in, 5 out]
                n538 = local write "run lab02-1"(w840) -> ()
                n539 = case shown="True" w840 {
                  tunnel: w846 -> [_ w882]
                  tunnel: w845 -> [_ w881]
                  tunnel: w843 -> [w848 w880]
                  tunnel: w844 -> [_ w879]
                  tunnel: w842 -> [_ w878]
                  tunnel: [w847 w877] -> w841
                  tunnel: w839 -> [_ w876]
                  tunnel: w838 -> [_ w875]
                  tunnel: w837 -> [_ w874]
                  frame False {
                    # "stop test"
                    n540 = stacked-sequence {
                      tunnel: w848 -> [w857 _]
                      tunnel: [w849 _] -> w847
                      frame #0 {
                        n541 = local read "DISP LAB02-1"() -> (w856:T4)
                        n542 = Unbundle(w856) -> ("CYCLE"=w854:dbl, "MINS"=w855:dbl)  [unwired: 1 out]
                        n543 = case shown="\"CYCLE TEST\"" w857 {
                          tunnel: w855 -> [_ _ w864]
                          tunnel: w854 -> [w862 w863 _]
                          tunnel: [w862 w863 w864] -> w853
                          frame "CHART TEST", Default {
                          }
                          frame "CYCLE TEST" {
                          }
                          frame "T-RISE TEST" {
                          }
                        }
                        n544 = local read "TDMS LAB02-1"() -> (w861:refnum<k34>)
                        n545 = Build Array("STOPPED") -> (w858:string[])
                        n546 = Build Array(w853) -> (w852:dbl[])
                        n547 = TDMS Write(0:w861, 5:"TEST RESULT", 7:w858, 9:w852) -> (4:w850:refnum<k34>, 15:w851:errorcluster)  [unwired: 2 in, 2 out]
                        n548 = TDMS Close(8:w851, 11:w850) -> (0:w849:errorcluster)  [unwired: 1 out]
                      }
                      frame #1 {
                        n549 = local read "DISP LAB02-1"() -> (w868:T4)
                        n550 = stacked-sequence {
                          tunnel: "LAB02-1" -> [w870 w872]
                          frame #0 {
                            n551 = call "sub vi - defrag tdms v1.vi"("panel id"=w870) -> ("error out"=w869:errorcluster)  [unwired: 10 in]
                            n552 = local write "data file error"(w869) -> ()
                          }
                          frame #1 {
                            n553 = local write "RESULT LAB02-1"(FALSE) -> ()
                            n554 = call "Save data file to network drive v2.vi"("panel id"=w872) -> ("network file save error"=w871:errorcluster)  [unwired: 9 in, 1 out]
                            n555 = local write "data file error"(w871) -> ()
                          }
                        }
                        n556 = Bundle(cluster=w868, "STATUS"="STOP") -> (w866:T4)  [unwired: 2 in]
                        n557 = local write "DISP LAB02-1"(w866) -> ()
                      }
                    }
                  }
                  frame True {
                    # "start new test and create test file"
                    n558 = stacked-sequence {
                      seq-local: [w883 _ _ _ _] -> [_ w907 _ _ _]
                      tunnel: w882 -> [w888 _ _ _ _]
                      tunnel: w881 -> [w885 _ _ _ _]
                      tunnel: w880 -> [w898 _ _ _ _]
                      tunnel: w879 -> [w891 _ _ _ _]
                      tunnel: w878 -> [w886 _ _ _ _]
                      tunnel: [_ w902 _ _ _] -> w877
                      tunnel: w876 -> [_ _ _ w928 _]
                      tunnel: w875 -> [_ _ _ w927 _]
                      tunnel: w874 -> [_ _ _ w926 _]
                      frame #0 {
                        w884 = "\\"
                        n559 = local read "SET LAB02-1"() -> (w893:T5)
                        n560 = case shown="\"CYCLE TEST\"" w898 {
                          tunnel: ["L02-1-CHART TEST-" "L02-1-CYCLE TEST-" "L02-1-T-RISE TEST-"] -> w894
                          frame "CHART TEST", Default {
                          }
                          frame "CYCLE TEST" {
                          }
                          frame "T-RISE TEST" {
                          }
                        }
                        n561 = Unbundle(w893) -> ("DESCRIPTION"=w892:string)  [unwired: 4 out]
                        n562 = Concatenate Strings(w888, "\\", w886, w884, w885, w884) -> (w895:string)
                        n563 = String To Path(string=w895) -> (path=w897:path)
                        n564 = Concatenate Strings(w895, w894, w892, "-", w891, ".tdms") -> (w883:string)
